vi "Execute.vi"(8 "error in":errorcluster, 11 "O3 Valve Step in":refnum<class "Speaker Step.lvclass">) -> (0 "error out":errorcluster, 1 "Next Step?":bool, 2 "MSG":string, 3 "O3 Valve Step out":refnum<class "Speaker Step.lvclass">)   [LabVIEW 2017, in "Controller.lvlib" / "Speaker Step.lvclass"]
uses:
  Speaker Step.lvclass
  C:/Program Files (x86)/National Instruments/LabVIEW 2017/vi.lib/MSR Consulting, LLC/General Reuse/Sequence/STEPS/LEAVES/Switch/Switch Step.lvclass
  Messages/Forward Command/Forward Command MSG.lvclass
  C:/Program Files (x86)/National Instruments/LabVIEW 2017/vi.lib/ActorFramework/Message/Message.lvclass
  PAS/Commands/Change Speaker State Cmd/Change Speaker State CMD.lvclass
  C:/Program Files (x86)/National Instruments/LabVIEW 2017/vi.lib/MSR Consulting, LLC/General Reuse/PAS/Commands/Change Speaker State CMD/Change Speaker State CMD.lvclass
  C:/Program Files (x86)/National Instruments/LabVIEW 2017/vi.lib/MSR Consulting, LLC/General Reuse/Command/Command.lvclass
  Speaker Step.lvclass/Speaker Step.ctl
  <vilib>/MSR Consulting, LLC/General Reuse/PAS/Commands/Change Speaker State CMD/Change Speaker State CMD.lvclass/Change Speaker State CMD.ctl
  Messages/Forward Command/Forward Command MSG.lvclass/Forward Command MSG.ctl
  <vilib>/ActorFramework/Message Enqueuer/Message Enqueuer.lvclass/Message Enqueuer.ctl
  <vilib>/MSR Consulting, LLC/General Reuse/PAS/Commands/Change Speaker State CMD/Write state.vi
  <vilib>/MSR Consulting, LLC/General Reuse/PAS/Commands/Change Speaker State CMD/Write cell.vi
  Read cell.vi
  Messages/Forward Command/Write id.vi
  Messages/Forward Command/Write CMD.vi
  <vilib>/ActorFramework/Message Priority Queue/Priority Enqueue.vi
  gController.lvclass
  <vilib>/ActorFramework/Message Enqueuer/Message Enqueuer.lvclass
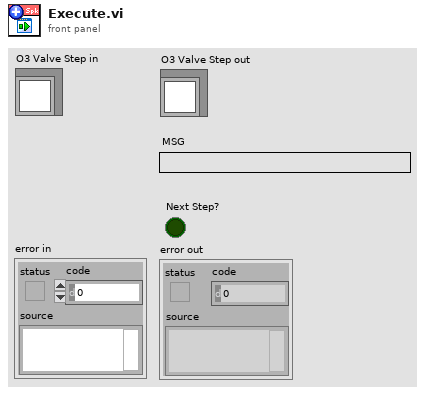
[diagram p1: front panel]
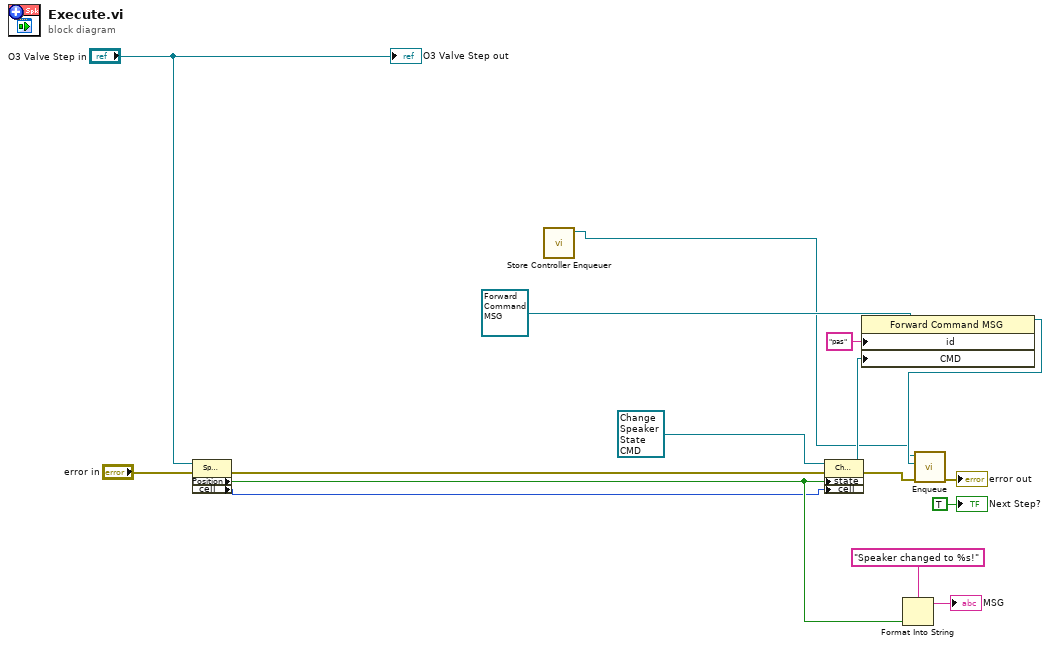
[diagram p0: block diagram]
diagram:
  n1 = property class="Speaker Step"(reference="O3 Valve Step in", error in="error in") -> (error out=w14:errorcluster, "Position"=w9:bool, "cell"=w1:u8)  [unwired: 1 out]
  n2 = call "Store Controller Enqueuer.vi"() -> ("Controller Enqueuer Out"=w2:refnum<class "Message Enqueuer.lvclass">)  [unwired: 11 in]
  n3 = property class="Change Speaker State CMD"(reference=refnum<class "Change Speaker State CMD.lvclass"> refnum ("gPAS Library.lvlib:Change Speaker State CMD"), error in=w14, "state"=w9, "cell"=w1) -> (reference out=w4:refnum<class "Change Speaker State CMD.lvclass">, error out=w13:errorcluster)
  n4 = property class="Forward Command MSG"(reference=refnum<class "Forward Command MSG.lvclass"> refnum ("Controller.lvlib:Forward Command MSG"), "id"="pas", "CMD"=w4) -> (reference out=w3:refnum<class "Forward Command MSG.lvclass">)  [unwired: 1 in, 1 out]
  n5 = Format Into String(format string="Speaker changed to %s!" ("MSG 2"), w9) -> (resulting string=→"MSG":string)  [unwired: 2 in, 1 out]
  n6 = call <vilib>:"Enqueue.vi"("error in (no error)"=w13, "Message"=w3, "Message Enqueuer in"=w2) -> ("error out"=→"error out":errorcluster)  [unwired: 7 in, 1 out]
  "O3 Valve Step out" <- "O3 Valve Step in"
  "Next Step?" <- TRUE ("Next Step?")
